vi "MALT Output Set One.vi"(6 "MALT FamilyCode":T1=enum."MALT132", 7 "error in":errorcluster, 8 "State":bool, 9 "Relay Num":i32, 10 "Address":i32) -> (0 "error out":errorcluster)   [LabVIEW 2018, in "AltonTech MALT200817.lvlib"]
uses:
  <instrlib>/AltonTech MALT/AltonTech MALT200817.lvlib
  <instrlib>/AltonTech MALT/Public/Types/MALT Family Codes.ctl
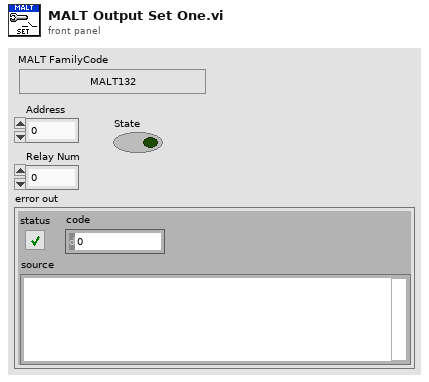
[diagram p1: front panel]
types:
  T1 = typedef "AltonTech MALT200817.lvlib/MALT Family Codes.ctl" = enum32{"-", "MALT40IO", "YAV904X8", "MALT132", "YAV91616", "MALT16PIN", "YAV90096", "YAV90HVT", "YAV90CLR", "YAV90128", "YAV90PNE", "YAVCANCON", "YAV91775", "YAV90XXX", "YAV90MMU", "H730050", "H710060", "H710061", "YAV90304", "MMI", "YAV90060", "MALT160T", "YAV90059", "Not Defined"}
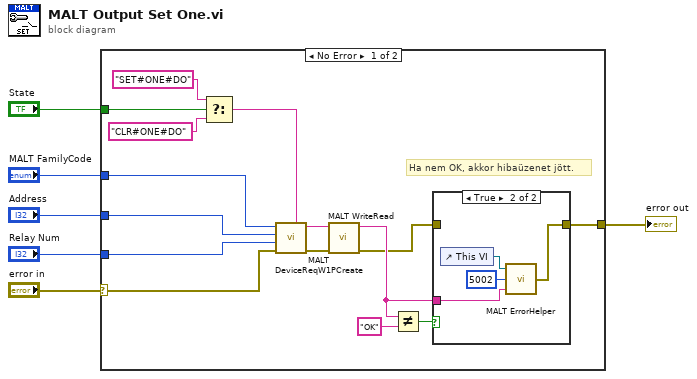
[diagram p0: block diagram]
diagram:
  n1 = case shown="No Error" "error in" {
    selector: "error in" -> [w8 w27]
    tunnel: "Address" -> [w19 _]
    tunnel: "MALT FamilyCode" -> [w18 _]
    tunnel: [w14 w27] -> w4
    tunnel: "State" -> [w12 _]
    tunnel: "Relay Num" -> [w7 _]
    frame No Error {
      # "Ha nem OK, akkor hibaüzenet jött."
      n2 = Select(t="SET#ONE#DO" ("cmd"), s=w12, f="CLR#ONE#DO" ("cmd")) -> (s? t:f=w9:string)
      n3 = call <instrlib>:"MALT DeviceReqW1PCreate.vi"("Cmd"=w9, "error in"=w8, "Param1"=w7, "Address"=w19, "FamilyCode"=w18) -> ("error out"=w20:errorcluster, "Request"=w21:string)  [unwired: 4 in]
      n4 = call <instrlib>:"MALT WriteRead.vi"("error in"=w20, "Request"=w21) -> ("error out"=w13:errorcluster, "Response"=w15:string)  [unwired: 8 in]
      n5 = Not Equal?(x=w15, y="OK") -> (x != y?=w16:bool)
      n6 = case shown="True" w16 {
        tunnel: w15 -> [_ w24]
        tunnel: [w22 w23] -> w14
        tunnel: w13 -> [w22 _]
        frame False {
        }
        frame True {
          n7 = control-ref of="This VI"() -> (w26:refnum<vi>)
          n8 = call <instrlib>:"MALT ErrorHelper.vi"("Message"=w24, "Code"=5002, "This VI"=w26) -> ("error out"=w23:errorcluster)
        }
      }
    }
    frame Error {
    }
  }
  "error out" <- w4
